vi "SearchForAddons.vi"(8 "error in (no error)":errorcluster, 11 "UIManager in":refnum<class "UIManager.lvclass">) -> (0 "error out":errorcluster, 3 "UIManager out":refnum<class "UIManager.lvclass">)   [LabVIEW 2020, in "UserInterface.lvlib" / "UIManager.lvclass"]
uses:
  UIManager.lvclass
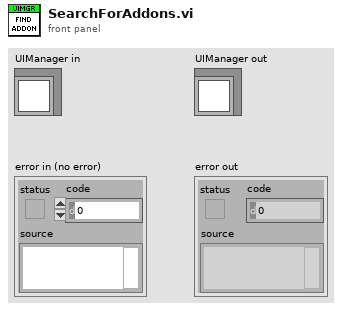
[diagram p1: front panel]
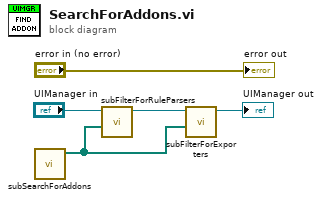
[diagram p0: block diagram]
diagram:
  n1 = call "subSearchForAddons.vi"() -> ("Addons"=w1:path[])  [unwired: 11 in]
  n2 = call "subFilterForRuleParsers.vi"("Addons"=w1, "UIManager in"="UIManager in") -> ("UIManager out"=w3:refnum<class "UIManager.lvclass">)  [unwired: 8 in, 1 out]
  n3 = call "subFilterForExporters.vi"("Addons"=w1, "UIManager in"=w3) -> ("UIManager out"=→"UIManager out":refnum<class "UIManager.lvclass">)  [unwired: 8 in, 1 out]
  "error out" <- "error in (no error)"
